vi "SetItemsVisible.vi"(8 "error in (no error)":errorcluster, 10 "Visibility Cluster":T1={"Hierarchy Lines"=enum."Visible", "Symbols"=TRUE, "Column Headers"=FALSE, "Row Headers"=FALSE, "Horizontal Lines"=FALSE, "Vertical Lines"=FALSE}, 11 "Tree_LVOOP in":refnum<class "Tree Class.lvclass">) -> (0 "error out":errorcluster, 3 "Tree_LVOOP out":refnum<class "Tree Class.lvclass">)   [LabVIEW 2012, in "Tree Tools.lvlib" / "Tree Class.lvclass"]
uses:
  Tree Class.lvclass
  Tree Class.lvclass/Tree Class.ctl
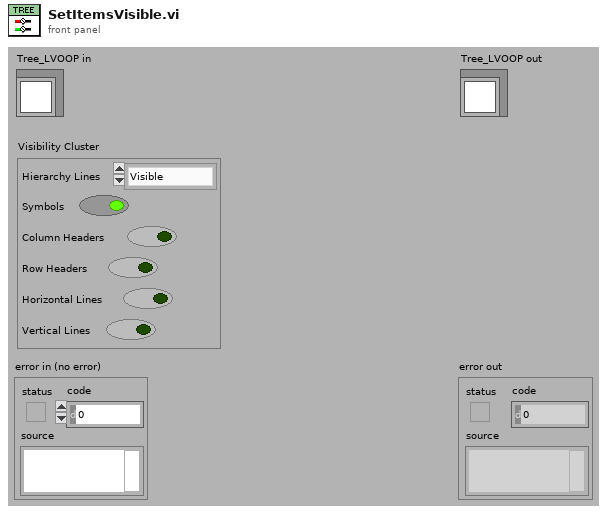
[diagram p1: front panel]
types:
  T1 = cluster{"Hierarchy Lines":enum32{"Visible", "Invisible", "OS Default"}, "Symbols":bool, "Column Headers":bool, "Row Headers":bool, "Horizontal Lines":bool, "Vertical Lines":bool}
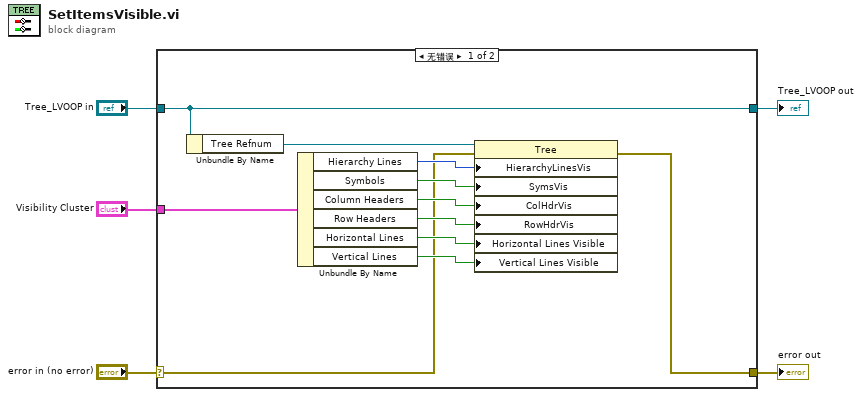
[diagram p0: block diagram]
diagram:
  n1 = case shown="无错误" "error in (no error)" {
    selector: "error in (no error)" -> [w7 w18]
    tunnel: [w6 w18] -> w4
    tunnel: [w16 w17] -> w2
    tunnel: "Tree_LVOOP in" -> [w16 w17]
    tunnel: "Visibility Cluster" -> [w14 _]
    frame No Error {
      n2 = Unbundle By Name(w16) -> ("Tree Refnum"=w15:refnum<vi>)
      n3 = Unbundle By Name(w14) -> ("Hierarchy Lines"=w13:enum32{"Visible", "Invisible", "OS Default"}, "Symbols"=w12:bool, "Column Headers"=w11:bool, "Row Headers"=w10:bool, "Horizontal Lines"=w9:bool, "Vertical Lines"=w8:bool)
      n4 = property class="Tree"(reference=w15, error in=w7, "HierarchyLinesVis"=w13, "SymsVis"=w12, "ColHdrVis"=w11, "RowHdrVis"=w10, "Horizontal Lines Visible"=w9, "Vertical Lines Visible"=w8) -> (error out=w6:errorcluster)  [unwired: 1 out]
    }
    frame Error {
    }
  }
  "error out" <- w4
  "Tree_LVOOP out" <- w2
